vi "extractADCData.vi"(8 "error in (no error)":errorcluster, 11 "Model in":refnum<class "Model.lvclass">) -> (0 "error out":errorcluster, 3 "Model out":refnum<class "Model.lvclass">)   [LabVIEW 2012, in "Model.lvclass"]
uses:
  Model.lvclass
  Model.lvclass/Model.ctl
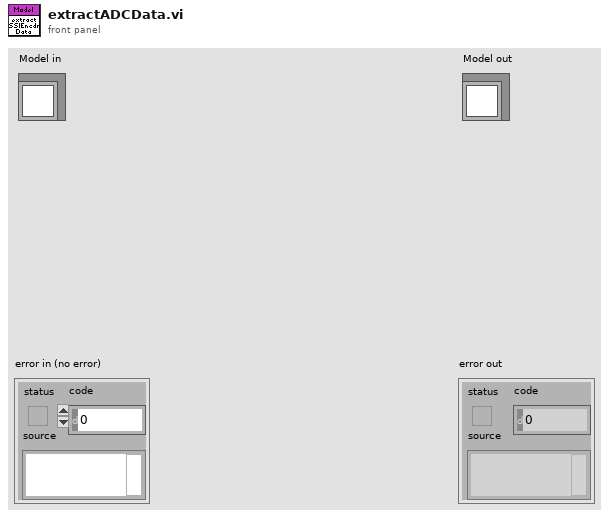
[diagram p1: front panel]
types:
  T1 = typedef "ILCCommon.lvlib/ILCConfiguration.lvlib/InputChannels.ctl" = enum16{"Channel 0", "3 Channels", "5 Channels"}
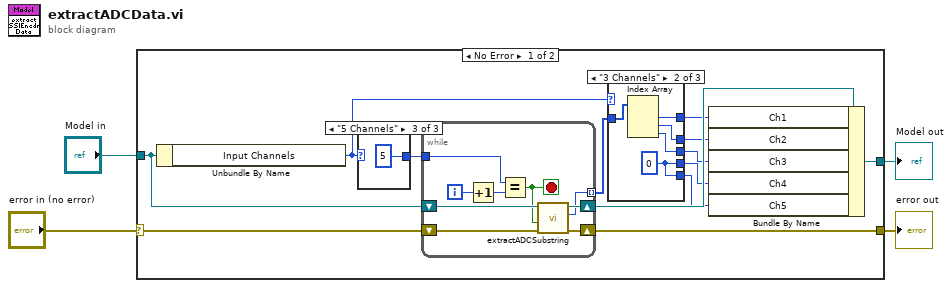
[diagram p0: block diagram]
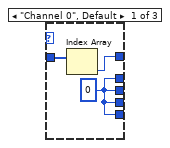
[diagram p2: hidden frame]
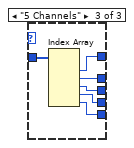
[diagram p3: hidden frame]
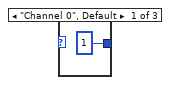
[diagram p4: hidden frame]
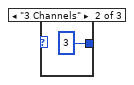
[diagram p5: hidden frame]
diagram:
  n1 = case shown="No Error" "error in (no error)" {
    selector: "error in (no error)" -> [w13 w45]
    tunnel: [w5 w45] -> w3
    tunnel: [w16 w44] -> w1
    tunnel: "Model in" -> [w15 w44]
    frame No Error {
      n2 = Unbundle By Name(w15) -> ("Input Channels"=w12:T1)
      n3 = case shown="\"5 Channels\"" w12 {
        tunnel: [1 3 5] -> w14
        frame "Channel 0", Default {
        }
        frame "3 Channels" {
        }
        frame "5 Channels" {
        }
      }
      n4 = while {
        tunnel: w14 -> [w39]
        tunnel: [w37] -> w11 mode=indexing
        shift-right: [w36] -> w5
        shift-left: w13 -> [w35]
        shift-right: [w43] -> w17
        shift-left: w15 -> [w42]
        i -> [w41]
        stop <- w38 stop-if-true
        n5 = Increment(x=w41) -> (x+1=w40:i32)
        n6 = Equal?(x=w39, y=w40) -> (x = y?=w38:bool)
        n7 = call "extractADCSubstring.vi"("error in (no error)"=w35, "lastIsTrue?"=w38, "Model in"=w42) -> ("error out"=w36:errorcluster, "adcElement"=w37:i32, "Model out"=w43:refnum<class "Model.lvclass">)  [unwired: 6 in]
      }
      n8 = case shown="\"3 Channels\"" w12 {
        tunnel: w11 -> [w20 w25 w31]
        tunnel: [w19 w23 w30] -> w10
        tunnel: [w18 w21 w26] -> w9
        tunnel: [w18 w22 w29] -> w8
        tunnel: [w18 w24 w28] -> w7
        tunnel: [w18 w24 w27] -> w6
        frame "Channel 0", Default {
          w18 = 0 ("InputData.ADCs.Ch2")
          n9 = Index Array(array=w20) -> (element=w19:i32)  [unwired: 1 in]
        }
        frame "3 Channels" {
          w24 = 0 ("InputData.ADCs.Ch2")
          n10 = Index Array(array=w25) -> (element #1=w23:i32, element #2=w21:i32, element #3=w22:i32)  [unwired: 3 in]
        }
        frame "5 Channels" {
          n11 = Index Array(array=w31) -> (element #1=w30:i32, element #2=w26:i32, element #3=w29:i32, element #4=w28:i32, element #5=w27:i32)  [unwired: 5 in]
        }
      }
      n12 = Bundle By Name(cluster=w17, "Ch1"=w10, "Ch2"=w9, "Ch3"=w8, "Ch4"=w7, "Ch5"=w6) -> (w16:refnum<class "Model.lvclass">)
    }
    frame Error {
    }
  }
  "error out" <- w3
  "Model out" <- w1
